vi "PH_Stepmotor_BaseClass.destructor.vi"(0 "i ref in":refnum<vi>, 5 "error in":errorcluster) -> (19 "error out":errorcluster)   [LabVIEW 2014, in "PH_Stepmotor_BaseClass.lvlib"]
doc: "This is the destructor of a class.\n\nLicense Agreement for this software:\n\nCopyright (C)\nGesellschaft für Schwerionenforschung, GSI\nPlanckstr. 1\n64291 Darmstadt\nGermany\n\nContact: D.Beck@gsi.de \n\nThis program is free software; you can redistribute it and/or modify it under the terms of the \nGNU General Public License as published by the Free Software Foundation; either version 2 of \nthe license, or (at your option) any later version.\n\nThis program is distributed in the hope that it will be useful, but WITHOUT ANY WARRANTY; \nwithout even the implied warranty of MERCHANTABILITY or FITNESS FOR A PARTICULAR PURPOSE. See the GNU General License for more details (http://www.gnu.org).\n\nGesellschaft für Schwerionenforschung, GSI\nPlanckstr. 1, 64291 Darmstadt, Germany\nFor all questions and ideas contact: M.Richter@gsi.de, H.Brand@gsi.de or D.Beck@gsi.de.\nLast update: 16-JUN-2004"
uses:
  PH_Stepmotor_BaseClass.lvlib
  CSlibraries-extern/DimLVEvent/LVDimInterface/LVDimInterface.lvlib
  CS_Core/CSSystem/CSSystemLib/CSSystemLib.lvlib
  PH_PSDBWriter/PH_PSDBWriter.lvlib
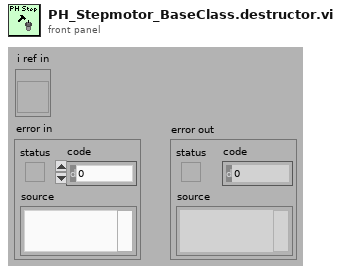
[diagram p1: front panel]
types:
  T1 = typedef "PH_Stepmotor_BaseClass.lvlib/PH_Stepmotor_BaseClass.i attribute.ctl" = cluster{"Device Error":errorcluster, "Axes PSDB Thread":cluster{"Ref":refnum<vi>, "Q-Ref":refnum<queue>, "Data Status":T2}, "Axes":T3[], "Axes PSDB Infos":cluster{"GUI Name":string, "PSDB Instance ID":i32, "PSDB Status Service ID":i32, "Axis":i32, "Class":string}[], "GUI Refs":T8}
  T2 = typedef "PH_PSDBWriter.lvlib/PH_PSDBWriter.Data Status.ctl" = i16
  T3 = typedef "PH_Stepmotor_BaseClass.lvlib/PH_Stepmotor_BaseClass.Axis Attributes.ctl" = cluster{"Settings":T4, "Endswitch?":bool, "DIM Service IDs":T6, "Activity":T7, "Configured?":bool, "Position":cluster{"Current":i32, "Target":i32}, "Position to set":cluster{"New?":bool, "Wanted":i32}, "Stop?":bool, "Reset?":bool, "Move?":bool, "Nothing connected?":bool}
  T4 = typedef "PH_Stepmotor_BaseClass.lvlib/PH_Stepmotor_BaseClass.Axis Settings.ctl" = cluster{"Sign change":bool, "Width":dbl, "Calibration":dbl, "Unit":string, "Motor Type":T5, "Unit Width":string, "Unit CF":string}
  T5 = typedef "PH_Stepmotor_BaseClass.lvlib/PH_Stepmotor_BaseClass.Motor Type.ctl" = enum16{"Unspecific", "OWIS 49.120.2633", "OWIS 49.060.1033", "OWIS 43.040.2558", "Diamond Motion 2200 series", "OWIS 49.120.266B.MV6", "Calorimeter", "Linear Stage 1", "MICOS VT-80", "MICOS VT-80 S", "Standa Rotstage nt0.95A", "PUF RA 320.200", "PUF RA 800.200", "PUF RA 800.400", "PUF RA 400.50", "1324.nn.800.50", "1324.n9c.800.50", "1324.nn.320.200", "1324.nn.400.200", "1324.nn.800.200", "1324.nn.400.50", "1324.8c9c.800.50", "1324.8c9c.400.200"}
  T6 = typedef "PH_Stepmotor_BaseClass.lvlib/PH_Stepmotor_BaseClass.Axis DIM Service IDs.ctl" = cluster{"Settings":i32, "Information":i32}
  T7 = typedef "PH_Stepmotor_BaseClass.lvlib/PH_Stepmotor_BaseClass.Axis Activity.ctl" = enum16{"No Information", "stopped", "running", "Failure", "Alarm", "stopped at backward ES", "stopped at foreward ES"}
  T8 = typedef "PH_Stepmotor_BaseClass.lvlib/PH_Stepmotor_BaseClass.GUI Refs.ctl" = cluster{"Axes Configuration":refnum<vi>, "Device Error":refnum<vi>, "Axes PSDB Infos":refnum<vi>}
  T9 = enum16{"SetAttribute", "GetAttribute", "CreateAttribute", "DestroyAttribute", "DestroyAllAtributes"}
  T10 = cluster{"GUI Name":string, "PSDB Instance ID":i32, "PSDB Status Service ID":i32, "Axis":i32, "Class":string}[]
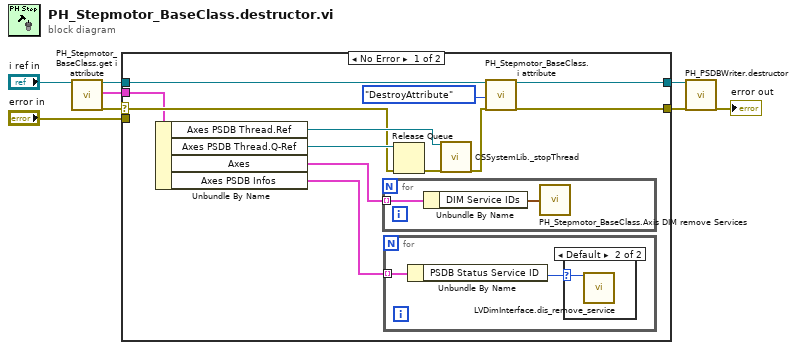
[diagram p0: block diagram]
diagram:
  n1 = call "PH_Stepmotor_BaseClass.get i attribute.vi"("i ref in"="i ref in") -> ("i ref out"=w7:refnum<vi>, "i attribute"=w1:T1, "error out"=w6:errorcluster)  [unwired: 16 in]
  n2 = case shown="No Error" w6 {
    selector: w6 -> [w10 _]
    tunnel: [w12 w26] -> w5
    tunnel: w7 -> [w11 w27]
    tunnel: [w13 w27] -> w3
    tunnel: "error in" -> [_ w26]
    tunnel: w1 -> [w9 _]
    frame No Error {
      n3 = Unbundle By Name(w9) -> ("Axes PSDB Thread.Ref"=w20:refnum<vi>, "Axes PSDB Thread.Q-Ref"=w19:refnum<queue>, "Axes"=w15:T3[], "Axes PSDB Infos"=w16:T10)
      n4 = for {
        tunnel: w15 -> [w25] mode=indexing
        n5 = Unbundle By Name(w25) -> ("DIM Service IDs"=w24:T6)
        n6 = call "PH_Stepmotor_BaseClass.Axis DIM remove Services.vi"("IDs"=w24) -> ()
      }
      n7 = for {
        tunnel: w16 -> [w22] mode=indexing
        n8 = Unbundle By Name(w22) -> ("PSDB Status Service ID"=w21:i32)
        n9 = case shown="Default" w21 {
          selector: w21 -> [_ w23]
          frame -1 {
          }
          frame Default {
            n10 = call "LVDimInterface.dis_remove_service.vi"("my_serviceID"=w23) -> ()  [unwired: 18 in, 1 out]
          }
        }
      }
      n11 = Release Queue(queue=w19, error in (no error)=w10) -> (error out=w17:errorcluster)  [unwired: 1 in, 2 out]
      n12 = call "CSSystemLib._stopThread.vi"("i ref in"=w20, "error in (no error)"=w17) -> ("error out"=w18:errorcluster)  [unwired: 16 in, 1 out]
      n13 = call "PH_Stepmotor_BaseClass.i attribute.vi"("VI Refnum"=w11, "Action"=T9."DestroyAttribute", "error in (no error)"=w18) -> ("VI Refnum out"=w13:refnum<vi>, "error out"=w12:errorcluster)  [unwired: 14 in, 1 out]
    }
    frame Error {
    }
  }
  n14 = call "PH_PSDBWriter.destructor.vi"("i ref in"=w3, "error in(no error)"=w5) -> ("error out"=→"error out":errorcluster)  [unwired: 17 in]
